vi "Cell Set Sink Current.vi"(7 "Box ID":u8=1, 8 "error in (no error)":errorcluster, 9 "Sink Current Limit (mA)":dbl, 10 "Channel":u16, 11 "CAN in":refnum<class "XNET_BS120x.lvclass">) -> (0 "error out":errorcluster, 3 "CAN out":refnum<class "XNET_BS120x.lvclass">)   [LabVIEW 2021, in "BS120x Driver.lvlib" / "XNET_BS120x.lvclass"]
uses:
  XNET_BS120x.lvclass
  BS120x.lvclass
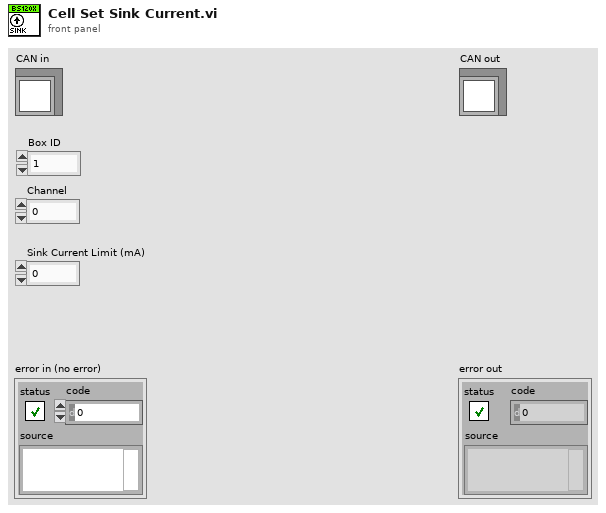
[diagram p1: front panel]
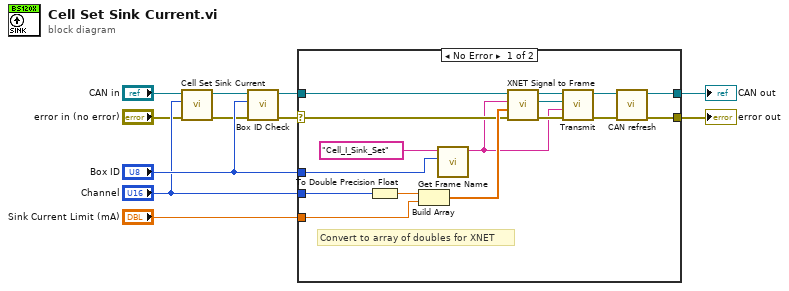
[diagram p0: block diagram]
diagram:
  n1 = call-parent "Cell Set Sink Current.vi"("error in (no error)"="error in (no error)", "Channel"="Channel", "BS120x in"="CAN in") -> ("error out"=w3:errorcluster, "BS120x out"=w4:refnum<class "XNET_BS120x.lvclass">)  [unwired: 7 in]
  n2 = call "Box ID Check.vi"("error in (no error)"=w3, "Box ID"="Box ID", "CAN in"=w4) -> ("error out"=w5:errorcluster, "CAN out"=w7:refnum<class "XNET_BS120x.lvclass">)  [unwired: 7 in]
  n3 = case shown="No Error" w5 {
    selector: w5 -> [w13 w29]
    tunnel: "Channel" -> [w26 _]
    tunnel: "Sink Current Limit (mA)" -> [w25 _]
    tunnel: w7 -> [w23 w28]
    tunnel: [w18 w29] -> w9
    tunnel: [w16 w28] -> w8
    tunnel: "Box ID" -> [w14 _]
    frame No Error {
      # "Convert to array of doubles for XNET"
      n4 = To Double Precision Float(number=w26) -> (double precision float=w27:dbl)
      n5 = Build Array(w27, w25) -> (w24:dbl[])
      n6 = call "Get Frame Name.vi"("Box ID"=w14, "Frame Name"="Cell_I_Sink_Set" ("Frame")) -> ("Frame Name out"=w12:string)  [unwired: 9 in]
      n7 = call "XNET Signal to Frame.vi"("error in (no error)"=w13, "Data Array"=w24, "Frame"=w12, "CAN in"=w23) -> ("error out"=w20:errorcluster, "Data"=w21:refnum<class "XNET Data.lvclass">, "CAN out"=w22:refnum<class "XNET_BS120x.lvclass">)  [unwired: 5 in]
      n8 = call "Transmit.vi"("error in (no error)"=w20, "Frame"=w12, "Data in"=w21, "CAN in"=w22) -> ("error out"=w19:errorcluster, "CAN out"=w17:refnum<class "XNET_BS120x.lvclass">)  [unwired: 6 in]
      n9 = call "CAN refresh.vi"("error in (no error)"=w19, "CAN in"=w17) -> ("error out"=w18:errorcluster, "CAN out"=w16:refnum<class "XNET_BS120x.lvclass">)  [unwired: 8 in]
    }
    frame Error {
    }
  }
  "error out" <- w9
  "CAN out" <- w8
